vi "PicoScope4000aExampleBlock.vi"() -> ()   [LabVIEW 2010]
doc: "This example demonstrates how to use the PicoScope Labview library to collect data using block mode."
uses:
  shared/PicoBuffers.ctl
  PicoScope4000aLib/PicoScope4000aAnalogChannelSettings.ctl
  shared/Buffer and Transfer Settings.ctl
  shared/Acquisition Settings.ctl
panel:
  out "Unit Info":T1
  in  "Resolution":u32(ring)=1 items=["8-bit", "12-bit", "14-bit"]
  in  "Trigger Settings":T2={"Trigger Enabled"=FALSE, "Trigger Source"=enum."Channel A", "Trigger Threshold (Volts/Probe units)"=0.0, "Trigger Direction"=2, "Trigger Delay (samples)"=0, "Auto Trigger Time (ms)"=1000} {"Trigger Direction" items=["Rising"=2, "Falling"=3]}
  out "overflow":i16 format="%08b"
  in  "Apply Settings":bool
  in  "Channel A Settings":T3={"Enabled"=TRUE, "Coupling"=1, "Range"=6, "Analogue Offset"=0.0, "Bandwidth Limit"=0} {"Bandwidth Limit" items=["Full", "20kHz", "100kHz", "1MHz"]; "Range" items=["10 mV", "20 mV", "50 mV", "100 mV", "200 mV", "500 mV", "1 V", "2 V", "5 V", "10 V", "20 V", "50 V ", "100 V"]; "Coupling" items=["AC", "DC"]}
  out "USB 3.0 device on non-USB 3.0 Port":bool=TRUE
  out "USB Powered":bool=TRUE
  out "error out":errorcluster
  in  "Data file":path=path "PicoScope4000aExampleBlock ChA Data"
  in  "Buffer and Transfer Settings":T4={"startIndex"=0, "Samples"=5000000, "Down Sample Ratio"=1, "Down-Sample Mode"=0} {"Down-Sample Mode" items=["RAW none"=2147483648, "None"=0, "Aggregate"=1, "Decimate"=2, "Average"=4]; "Down Sample Ratio" step=1; "Samples" format="%_6p"}
  in  "Acquisition Settings":T5={"preTriggerSamples"=0, "postTriggerSamples"=5000000, "timebase"=5} {"postTriggerSamples" format="%_6p"; "preTriggerSamples" format="%_6p"}
  out "Properties Panel":T6={"Sample Frequency"=41666668.0, "Sample Rate"=2.4000000209412065e-08, "Max Samples Available"=26843008, "Number of Samples"=0, "Total Capture Time (sec) "=0.0, "Max Total Capture Time Available (sec)"=0.6442322134971619} {"Max Total Capture Time Available (sec)" format="%.3p"; "Sample Frequency" format="%.6p"; "Sample Rate" format="%.3p"; "Max Samples Available" format="%_6p"; "Total Capture Time (sec)" format="%.3p"}
  in  "stop":bool
  out "Analog Channels":cluster{i32, dbl, "Data":dbl[]}[](graph)
  in  "Serial Number":string
  in  "Use Serial Number":bool
  in  "error in (no error)":errorcluster
  # "Bit 0 = ChA"
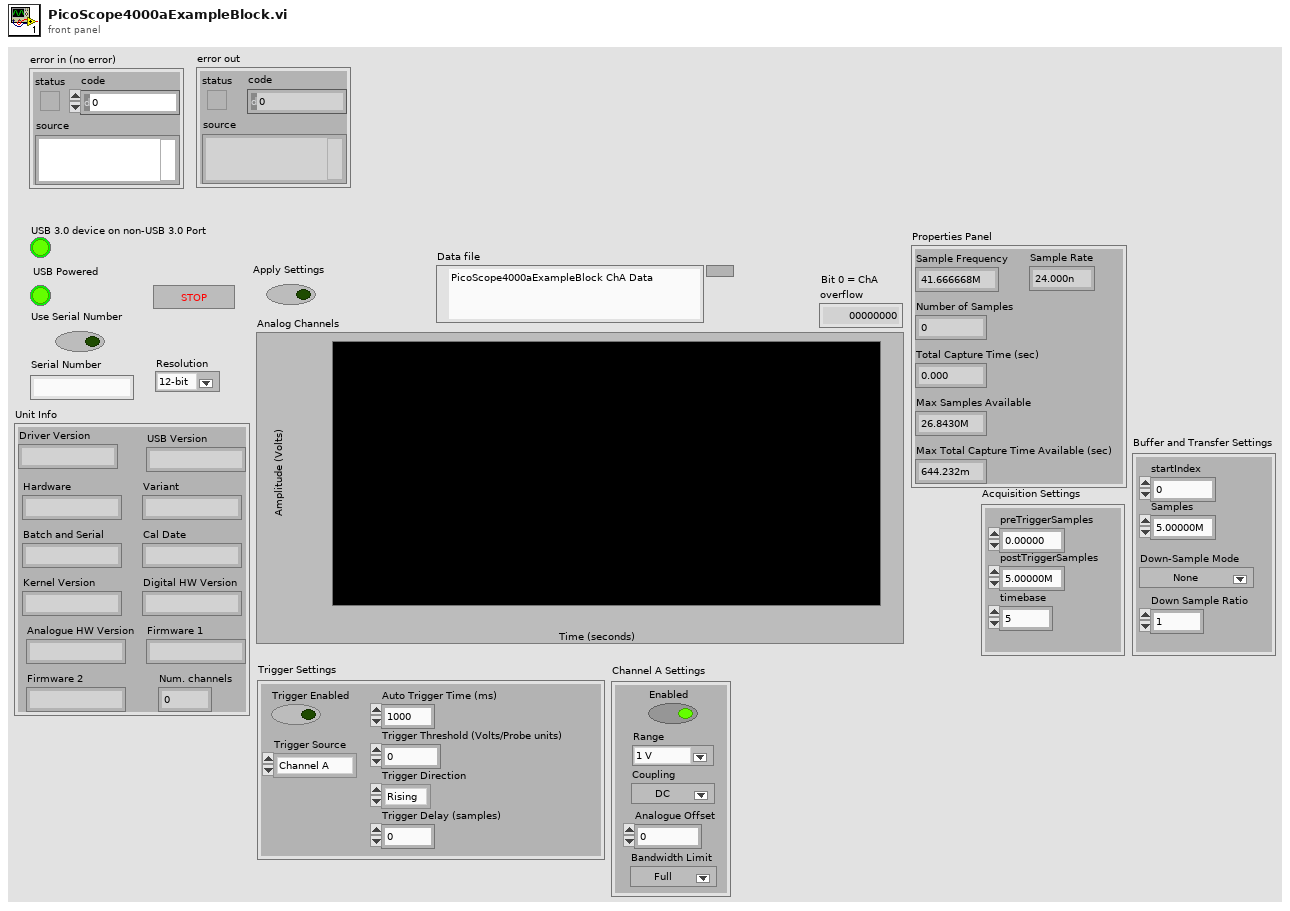
[diagram p1: front panel]
types:
  T1 = cluster{"Driver Version":string, "USB Version":string, "Hardware":string, "Variant":string, "Batch and Serial":string, "Cal Date":string, "Kernel Version":string, "Digital HW Version":string, "Analogue HW Version":string, "Firmware 1":string, "Firmware 2":string, "Num. channels":i16}
  T2 = cluster{"Trigger Enabled":bool, "Trigger Source":enum16{"Channel A", "Channel B", "Channel C", "Channel D", "Channel E", "Channel F", "Channel G", "Channel H"}, "Trigger Threshold (Volts/Probe units)":dbl, "Trigger Direction":u16, "Trigger Delay (samples)":u32, "Auto Trigger Time (ms)":i16}
  T3 = typedef "PicoScope4000aAnalogChannelSettings.ctl" = cluster{"Enabled":bool, "Coupling":i16, "Range":u16, "Analogue Offset":sgl, "Bandwidth Limit":u32}
  T4 = typedef "Buffer and Transfer Settings.ctl" = cluster{"startIndex":u64, "Samples":u64, "Down Sample Ratio":u64, "Down-Sample Mode":u32}
  T5 = typedef "Acquisition Settings.ctl" = cluster{"preTriggerSamples":u64, "postTriggerSamples":u64, "timebase":u32}
  T6 = cluster{"Sample Frequency":dbl, "Sample Rate":dbl, "Max Samples Available":u64, "Number of Samples":u64, "Total Capture Time (sec) ":dbl, "Max Total Capture Time Available (sec)":dbl}
  T7 = enum16{"open", "open or create", "create or replace", "create", "open (read-only)"}
  T8 = typedef "PicoBuffers.ctl" = cluster{"Max Buffer Pointers":u64[][][], "Min Buffer Pointers":u64[][][], "StreamingDataInfo":cluster{"Channel":u32, "Down-Sample Mode":u32, "PICO_DATA_TYPE":enum32{"PICO_INT8_T", "PICO_INT16_T", "PICO_INT32_T", "PICO_UINT32_T", "PICO_INT64_T", ""}, "Samples":i32, "bufferIndex":u64, "startIndex":i32, "overflow":i16}[][]}
  T9 = cluster{"Channel A Buffer":i16[], "Channel B Buffer":i16[], "Channel C Buffer":i16[], "Channel D Buffer":i16[], "Channel E Buffer":i16[], "Channel F Buffer":i16[], "Channel G Buffer":i16[], "Channel H Buffer":i16[], "Port 0 Buffer":i16[], "Port 1 Buffer":i16[]}[]
  T10 = cluster{"Channel A Buffer":i16[], "Channel B Buffer":i16[], "Channel C Buffer":i16[], "Channel D Buffer":i16[], "Channel E Buffer":i16[], "Channel F Buffer":i16[], "Channel G Buffer":i16[], "Channel H Buffer":i16[], "Port 0 Buffer":i16[], "Port 1 Buffer":i16[]}
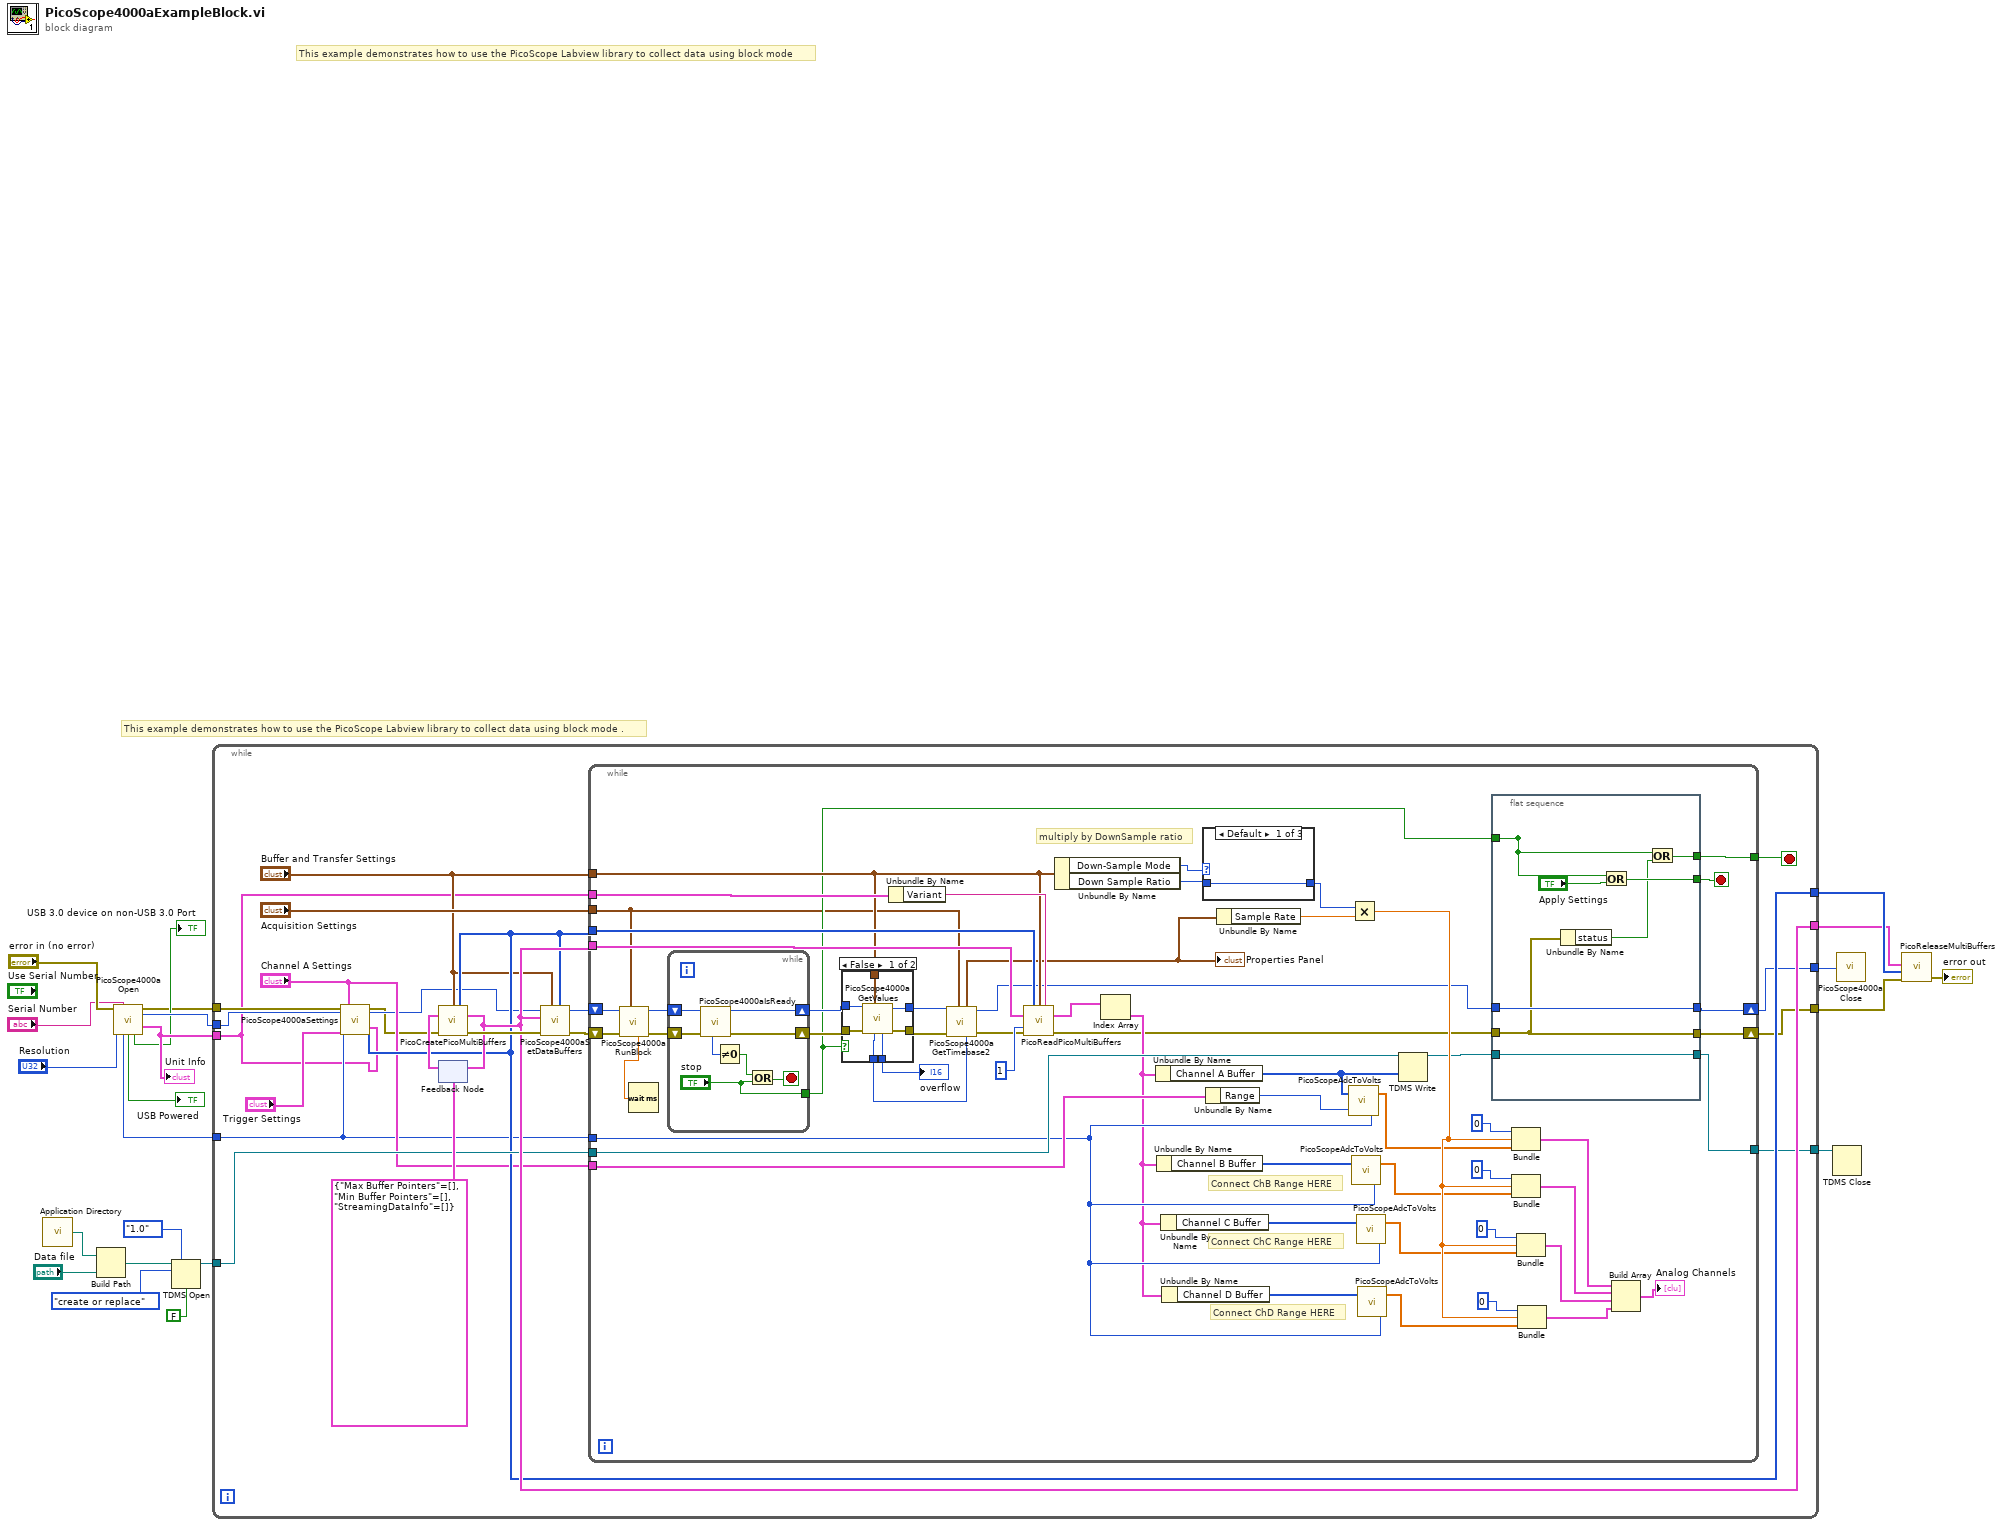
[diagram p0: block diagram]
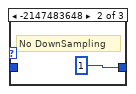
[diagram p3: hidden frame]
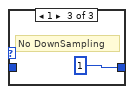
[diagram p4: hidden frame]
diagram:
  # "This example demonstrates how to use the PicoScope Labview library to collect data using block mode ."
  # "This example demonstrates how to use the PicoScope Labview library to collect data using block mode"
  n1 = call <vilib>:"Application Directory.vi"() -> ("Application Directory"=w15:path)
  n2 = Build Path(base path=w15, name or relative path="Data file") -> (appended path=w16:path)
  n3 = call "PicoScope4000aOpen.vi"("error in (no error)"="error in (no error)", "Serial Number"="Serial Number", "Resolution"="Resolution") -> ("error out"=w3:errorcluster, "handle"=w7:i16, "Unit Info"=w8:T1, "Max ADC value"=w11:i16, "USB powered"=→"USB Powered":bool, "USB 3.0 on non-USB 3.0 port"=→"USB 3.0 device on non-USB 3.0 Port":bool)  [unwired: 7 in]
  "Unit Info" <- w8
  n4 = TDMS Open(6:FALSE ("disable buffering? (T)"), 7:enum16{"1.0", "2.0"}."1.0" ("file format version (2.0)"), 10:T7."create or replace" ("operation (0:open)"), 11:w16) -> (3:w13:refnum<k34>)  [unwired: 2 in, 1 out]
  n5 = while {
    tunnel: w7 -> [w39]
    tunnel: w11 -> [w34]
    tunnel: [w37] -> w22
    tunnel: [w41] -> w21
    tunnel: [w32] -> w14
    tunnel: w13 -> [w40]
    tunnel: w3 -> [w38]
    tunnel: [w33] -> w10
    tunnel: [w30] -> w9
    tunnel: w8 -> [w23]
    stop <- w31 stop-if-true
    n6 = call "PicoScope4000aSettings.vi"("error in"=w38, "handle in"=w39, "Max ADC value"=w34, "Trigger Settings"="Trigger Settings", "Channel A Settings"="Channel A Settings", "Unit Info"=w23) -> ("error out"=w25:errorcluster, "handle out"=w26:i16, "Enabled array"=w37:i16[])  [unwired: 11 in]
    n7 = feedback #1(T8 {"Max Buffer Pointers"=[], "Min Buffer Pointers"=[], "StreamingDataInfo"=[]} ("Data Pointers")) -> (w43:T8)
    n8 = call "PicoCreatePicoMultiBuffers.vi"("Buffer and Transfer Settings"="Buffer and Transfer Settings", "enabled array"=w37, "Data Pointers In"=w43, "error in (no error)"=w25) -> ("Data Pointers"=w41:T8, "error out"=w42:errorcluster)  [unwired: 10 in]
    n9 = feedback-in #1(w41) -> ()
    n10 = call "PicoScope4000aSetDataBuffers.vi"("enabled array"=w37, "Buffer and Transfer Settings"="Buffer and Transfer Settings", "error in (no error)"=w42, "Data Pointers In"=w41, "handle in"=w26) -> ("error out"=w29:errorcluster, "handle out"=w28:i16)  [unwired: 5 in]
    n11 = while {
      tunnel: w41 -> [w101]
      tunnel: "Buffer and Transfer Settings" -> [w55]
      tunnel: w37 -> [w92]
      tunnel: "Channel A Settings" -> [w91]
      tunnel: "Acquisition Settings" -> [w46]
      tunnel: w34 -> [w90]
      tunnel: w23 -> [w87]
      tunnel: [w62] -> w31
      shift-right: [w66] -> w33
      shift-left: w29 -> [w56]
      shift-right: [w60] -> w30
      shift-left: w28 -> [w57]
      tunnel: w40 -> [w100]
      tunnel: [w64] -> w32
      stop <- w61 stop-if-true
      # "Connect ChB Range HERE"
      # "Connect ChD Range HERE"
      # "Connect ChC Range HERE"
      # "multiply by DownSample ratio"
      n12 = call "PicoScope4000aRunBlock.vi"("Acquisition Settings"=w46, "error in (no error)"=w56, "handle in"=w57) -> ("error out"=w94:errorcluster, "handle out"=w93:i16, "timeIndisposedMs"=w45:dbl)  [unwired: 5 in, 1 out]
      n13 = Wait (ms)(milliseconds to wait=w45) -> ()  [unwired: 1 out]
      n14 = while {
        shift-right: [w125] -> w58
        shift-left: w94 -> [w126]
        shift-right: [w124] -> w59
        shift-left: w93 -> [w123]
        tunnel: ["stop"] -> w54
        stop <- w120 stop-if-true
        n15 = call "PicoScope4000aIsReady.vi"("error in (no error)"=w126, "handle in"=w123) -> ("error out"=w125:errorcluster, "handle out"=w124:i16, "ready"=w122:i16)  [unwired: 7 in]
        n16 = Not Equal To 0?(x=w122) -> (x != 0?=w121:bool)
        n17 = Or(x=w121, y="stop") -> (x .or. y?=w120:bool)
      }
      n18 = case shown="False" w54 {
        tunnel: w58 -> [w108 w109]
        tunnel: w59 -> [w107 w110]
        tunnel: [w106 w110] -> w48
        tunnel: [w105 w109] -> w49
        tunnel: w55 -> [w104 _]
        tunnel: [w103 _] -> w53
        tunnel: [w102 _] -> w52
        frame False {
          n19 = call "PicoScope4000aGetValues.vi"("Buffer and Transfer Settings"=w104, "error in (no error)"=w108, "handle in"=w107) -> ("error out"=w105:errorcluster, "handle out"=w106:i16, "overflow"=w103:i16, "noOfSamples"=w102:u64)  [unwired: 5 in]
        }
        frame True {
        }
      }
      "overflow" <- w53
      n20 = Unbundle By Name(w87) -> ("Variant"=w88:string)
      n21 = call "PicoScope4000aGetTimebase2.vi"("Number of Samples"=w52, "Acquisition Settings"=w46, "error in (no error)"=w49, "handle in"=w48) -> ("error out"=w50:errorcluster, "handle out"=w47:i16, "Properties Panel"=w51:T6)  [unwired: 5 in]
      "Properties Panel" <- w51
      n22 = call "PicoReadPicoMultiBuffers.vi"("enabled array"=w92, "Buffer and Transfer Settings"=w55, "Variant"=w88, "Data Pointers"=w101, "No of Buffers"=1, "error in (no error)"=w50) -> ("MultiBuffers (Max or non-aggregated)"=w99:T9, "error out"=w63:errorcluster)  [unwired: 7 in, 1 out]
      n23 = Unbundle By Name(w55) -> ("Down-Sample Mode"=w97:u32, "Down Sample Ratio"=w98:u64)
      n24 = Index Array(array=w99) -> (element=w67:T10)  [unwired: 1 in]
      n25 = Unbundle By Name(w67) -> ("Channel A Buffer"=w76:i16[])
      n26 = Unbundle By Name(w67) -> ("Channel B Buffer"=w82:i16[])
      n27 = Unbundle By Name(w67) -> ("Channel C Buffer"=w74:i16[])
      n28 = Unbundle By Name(w67) -> ("Channel D Buffer"=w70:i16[])
      n29 = case shown="Default" w97 {
        tunnel: [w127 u64 1 ("Down Sample Ratio") u64 1 ("Down Sample Ratio")] -> w95
        tunnel: w98 -> [w127 _ _]
        frame Default {
        }
        frame -2147483648 {
          # "No DownSampling"
        }
        frame 1 {
          # "No DownSampling"
        }
      }
      n30 = Unbundle By Name(w91) -> ("Range"=w84:u16)
      n31 = Unbundle By Name(w51) -> ("Sample Rate"=w89:dbl)
      n32 = call "PicoScopeAdcToVolts.vi"("Max_adc"=w90, "Range Index"=w84, "Data"=w76) -> ("Data"=w77:dbl[])
      n33 = Multiply(x=w95, y=w89) -> (x*y=w96:dbl)
      n34 = call "PicoScopeAdcToVolts.vi"("Max_adc"=w90, "Data"=w82) -> ("Data"=w81:dbl[])  [unwired: 1 in]
      n35 = call "PicoScopeAdcToVolts.vi"("Max_adc"=w90, "Data"=w74) -> ("Data"=w73:dbl[])  [unwired: 1 in]
      n36 = call "PicoScopeAdcToVolts.vi"("Max_adc"=w90, "Data"=w70) -> ("Data"=w69:dbl[])  [unwired: 1 in]
      n37 = TDMS Write(0:w100, 9:w76) -> (4:w65:refnum<k34>)  [unwired: 4 in, 3 out]
      n38 = flat-sequence {
        tunnel: [w118] -> w61
        tunnel: [w111] -> _
        tunnel: [w115] -> w62
        tunnel: w47 -> [w114]
        tunnel: [w114] -> w60
        tunnel: w63 -> [w113]
        tunnel: [w113] -> w66
        tunnel: [w112] -> w64
        tunnel: w65 -> [w112]
        tunnel: w54 -> [w111]
        frame #0 {
          n39 = Unbundle By Name(w113) -> ("status"=w116:bool)
          n40 = Or(x=w111, y="Apply Settings") -> (x .or. y?=w118:bool)
          n41 = Or(x=w111, y=w116) -> (x .or. y?=w115:bool)
        }
      }
      n42 = Bundle(0, w96, "Data"=w77) -> (w80:cluster{i32, dbl, "Data":dbl[]})  [unwired: 1 in]
      n43 = Bundle(0, w96, "Data"=w81) -> (w79:cluster{i32, dbl, "Data":dbl[]})  [unwired: 1 in]
      n44 = Bundle(0, w96, "Data"=w73) -> (w72:cluster{i32, dbl, "Data":dbl[]})  [unwired: 1 in]
      n45 = Bundle(0, w96, "Data"=w69) -> (w68:cluster{i32, dbl, "Data":dbl[]})  [unwired: 1 in]
      n46 = Build Array(w80, w79, w72, w68) -> (→"Analog Channels":cluster{i32, dbl, "Data":dbl[]}[])
    }
  }
  n47 = TDMS Close(11:w14) -> ()  [unwired: 1 in, 2 out]
  n48 = call "PicoScope4000aClose.vi"("handle"=w9) -> ()
  n49 = call "PicoReleaseMultiBuffers.vi"("error in (no error)"=w10, "Enabled array"=w22, "Data Pointers"=w21) -> ("error out"=→"error out":errorcluster)  [unwired: 8 in]
